vi "remove all keys per section.vi"(7 "section":string, 8 "error in (no error)":errorcluster, 11 "Refnum in":T1) -> (0 "error out":errorcluster, 3 "Refnum out":T1)   [LabVIEW 2024, in "API Config Files Management.lvlib"]
doc: "This function removes all keys from a specified section in a configuration .ini file, given the section name. The result in the .ini file is the section without any keys, but the section itself remains."
uses:
  API Config Files Management.lvlib
  <vilib>/Utility/config.llb/NI_LVConfig.lvlib
  <vilib>/Utility/config.llb/Config Data RefNum.ctl
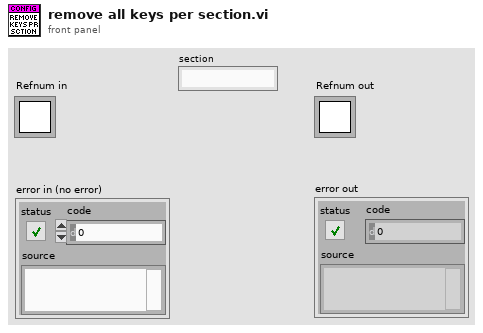
[diagram p1: front panel]
types:
  T1 = typedef "NI_LVConfig.lvlib/Config Data RefNum.ctl" = refnum<k1>
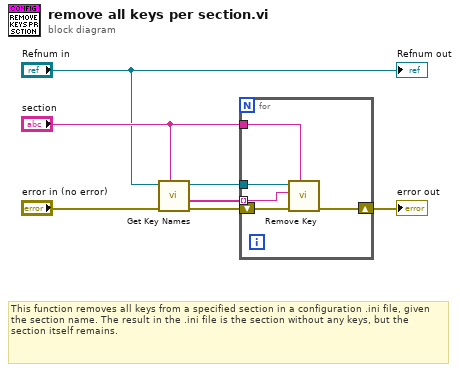
[diagram p0: block diagram]
diagram:
  # "This function removes all keys from a specified section in a configuration .ini file, given the section name. The result in the .ini file is the section without any keys, but the section itself remains."
  n1 = call <vilib>:"Get Key Names.vi"("section"="section", "error in (no error)"="error in (no error)", "refnum"="Refnum in") -> ("error out"=w4:errorcluster, "key names"=w5:string[], "refnum out"=w6:T1)  [unwired: 5 in, 1 out]
  n2 = for {
    tunnel: "section" -> [w12]
    tunnel: w6 -> [w10]
    tunnel: w5 -> [w9] mode=indexing
    shift-right: [w8] -> w1
    shift-left: w4 -> [w11]
    n3 = call <vilib>:"Remove Key.vi"("section"=w12, "error in (no error)"=w11, "key"=w9, "refnum"=w10) -> ("error out"=w8:errorcluster)  [unwired: 5 in, 2 out]
  }
  "error out" <- w1
  "Refnum out" <- "Refnum in"
